vi "SimpleGyroExample.vi"() -> ()   [LabVIEW 2014]
doc: "SimpleGyro Example\n\nThis example shows how to use a SimpleGyro sensor connected to the SPI port on the RoboRIO.\n\nThis example expects a USB cable connected from your development PC to the Type B USB Jack (next to the power input) on the roboRIO."
uses:
  <vilib>/Rock Robotics/SystemInterfaces/spilib/spi_bus.ctl
  SimpleGyro/SimpleGyro.lvlib
panel:
  in  "Reset Angle?":bool
  out "Device Found":bool
  in  "stop":bool
  out "Angle":dbl(knob) scale=0.0..360.0
  in  "SPI Chip Select":T1
  in  "Sample Rate (ms)":dbl=1.0 format="%#_13g"
  # "FRC Gyro & Accel Example"
  # "Gyro Configuration"
  # "FRC Gyro & Accel Placement"
  # "How to Install the FRC Gyro & Accel"
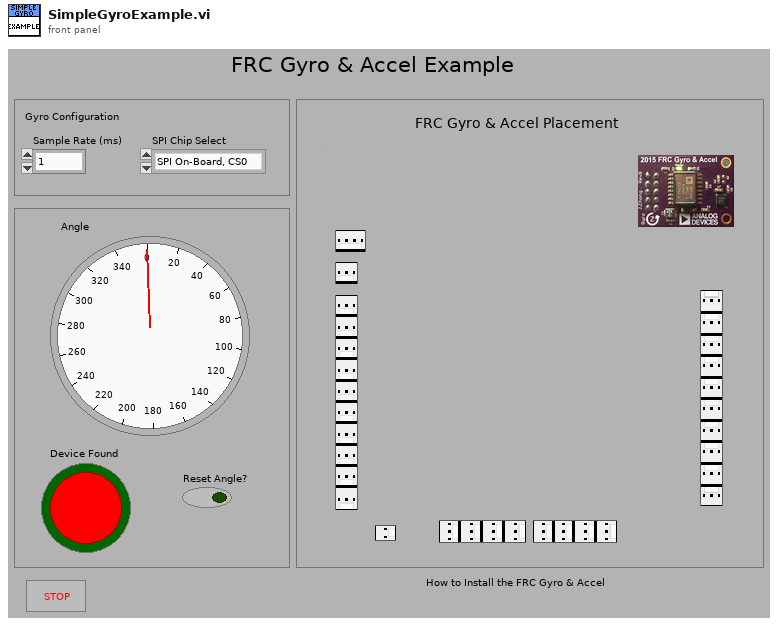
[diagram p1: front panel]
types:
  T1 = typedef "spi_bus.ctl" = enum16{"SPI On-Board, CS0", "SPI On-Board, CS1", "SPI On-Board, CS2", "SPI On-Board, CS3", "SPI MXP", "Invalid"}
  T2 = typedef "SimpleGyro.lvlib/WPI_SimpleGyroDevRef.ctl" = cluster{"DevStatus":errorcluster, "Handle":i32, "Controller":T3, "SPI Bus":T1, "Device Found":bool, "Sample Rate":dbl}
  T3 = typedef "FPGA_TypedefDigitalModule.ctl" = enum16{"Controller 1"}
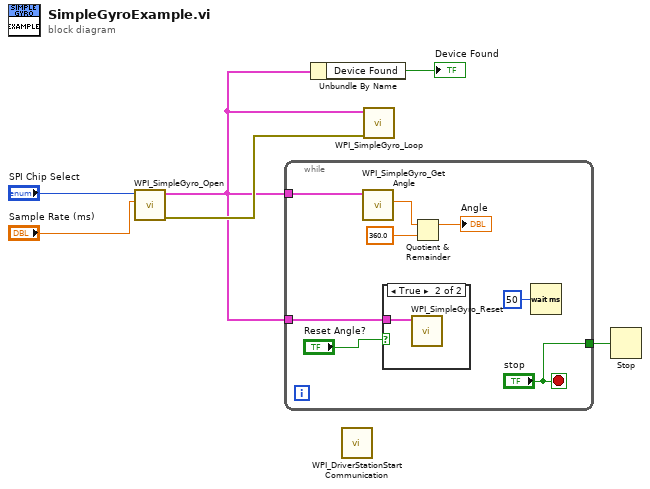
[diagram p0: block diagram]
diagram:
  n1 = call "WPI_SimpleGyro_Open.vi"("Sample Rate (ms)"="Sample Rate (ms)", "SPI Chip Select"="SPI Chip Select") -> ("error out"=w6:errorcluster, "SimpleGyroDevRef"=w1:T2)  [unwired: 8 in]
  n2 = while {
    tunnel: w1 -> [w7]
    tunnel: ["stop"] -> w3
    tunnel: w1 -> [w9]
    stop <- "stop" stop-if-true
    n3 = call "WPI_SimpleGyro_Get Angle.vi"("SimpleGyroDevRef"=w7) -> ("Angle"=w14:dbl)  [unwired: 8 in, 2 out]
    n4 = case shown="True" "Reset Angle?" {
      tunnel: w9 -> [_ w15]
      frame False {
      }
      frame True {
        n5 = call "WPI_SimpleGyro_Reset.vi"("SimpleGyroDevRef"=w15) -> ()  [unwired: 9 in, 2 out]
      }
    }
    n6 = Quotient & Remainder(x=w14, y=360.0) -> (x-y*floor(x/y)=→"Angle":dbl)  [unwired: 1 out]
    n7 = Wait (ms)(milliseconds to wait=u32 50) -> ()  [unwired: 1 out]
  }
  n8 = Unbundle By Name(w1) -> ("Device Found"=→"Device Found":bool)
  n9 = call <vilib>:"WPI_DriverStationStart Communication.vi"() -> ()  [unwired: 12 in]
  n10 = call "WPI_SimpleGyro_Loop.vi"("error in"=w6, "SimpleGyroDevRef"=w1) -> ()  [unwired: 9 in, 1 out]
  n11 = Stop(stop? (T)=w3) -> ()
